vi "Get All PDP Data.vi"(0 "Power Distribution Panel (0)":u8, 11 "error in":errorcluster) -> (6 "PDP Data":T1, 15 "error out":errorcluster)   [LabVIEW 2014]
doc: "Returns the currents of the Power Distribution Panel (PDP) channels."
uses:
  PDP Data.ctl
  <vilib>/Rock Robotics/WPI/CAN/PDP/WPI_CAN_PDPGlobalOps.ctl
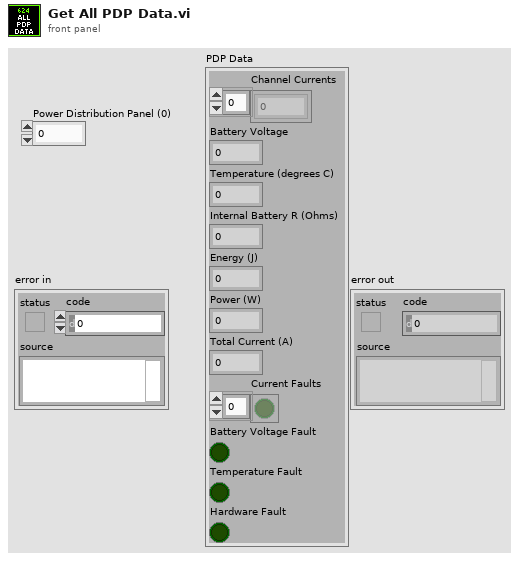
[diagram p1: front panel]
types:
  T1 = typedef "PDP Data.ctl" = cluster{"Channel Currents":dbl[], "Battery Voltage":dbl, "Temperature (degrees C)":dbl, "Internal Battery R (Ohms)":dbl, "Energy (J)":dbl, "Power (W)":dbl, "Total Current (A)":dbl, "Current Faults":bool[], "Battery Voltage Fault":bool, "Temperature Fault":bool, "Hardware Fault":bool}
  T2 = typedef "WPI_CAN_PDPGlobalOps.ctl" = enum16{"Write After Receive 0-5", "Write After Receive 6-11", "Write After Receive 12-15", "Write After Receive Energy", "Get All", "Get Commands", "Write Clear Sticky Faults Command", "Write Reset Energy Command", "Write Tare Currents Command", "Write Error", "Write After Receive Faults"}
  T3 = typedef "WPI_CAN_PDPGetAll.ctl" = cluster{"Channel Currents":dbl[], "Battery Voltage":dbl, "Temperature (degrees C)":dbl, "Internal Battery R (Ohms)":dbl, "Energy (J)":dbl, "Power (W)":dbl, "Total Current (A)":dbl, "CAN Error":errorcluster, "Current Faults":bool[], "Battery Voltage Fault":bool, "Temperature Fault":bool, "Hardware Fault":bool}
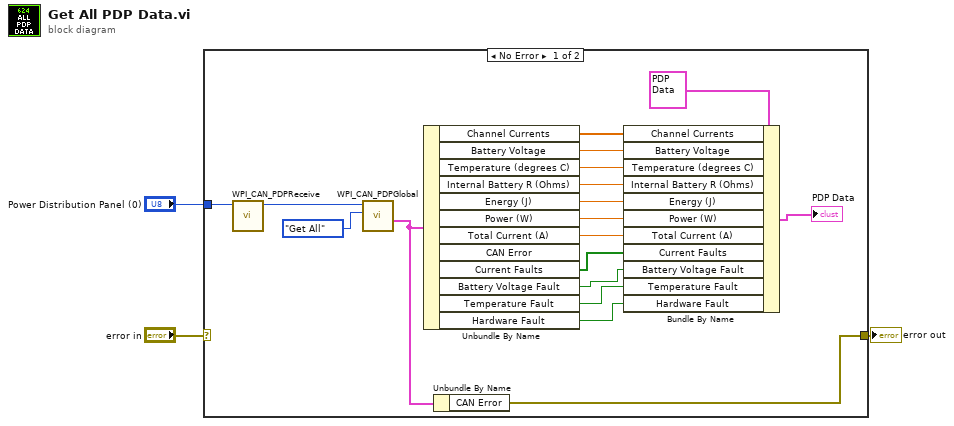
[diagram p0: block diagram]
diagram:
  n1 = case shown="No Error" "error in" {
    selector: "error in" -> [_ w22]
    tunnel: [w18 w22] -> w2
    tunnel: "Power Distribution Panel (0)" -> [w20 _]
    frame No Error {
      n2 = call <vilib>:"WPI_CAN_PDPReceive.vi"("Power Distribution Panel (0)"=w20) -> ("Power Distribution Panel Out"=w21:u8)  [unwired: 10 in]
      n3 = call <vilib>:"WPI_CAN_PDPGlobal.vi"("Operation"=WPI_CAN_PDPGlobalOps."Get All", "Power Distribution Panel (0)"=w21) -> ("Get All"=w17:T3)  [unwired: 7 in, 2 out]
      n4 = Unbundle By Name(w17) -> ("Channel Currents"=w14:dbl[], "Battery Voltage"=w13:dbl, "Temperature (degrees C)"=w12:dbl, "Internal Battery R (Ohms)"=w11:dbl, "Energy (J)"=w10:dbl, "Power (W)"=w9:dbl, "Total Current (A)"=w8:dbl, "Current Faults"=w7:bool[], "Battery Voltage Fault"=w6:bool, "Temperature Fault"=w5:bool, "Hardware Fault"=w4:bool)  [unwired: 1 out]
      n5 = Unbundle By Name(w17) -> ("CAN Error"=w18:errorcluster)
      n6 = Bundle By Name(cluster=T1 {"Channel Currents"=[], "Battery Voltage"=0.0, "Temperature (degrees C)"=0.0, "Internal Battery R (Ohms)"=0.0, "Energy (J)"=0.0, "Power (W)"=0.0, "Total Current (A)"=0.0, "Current Faults"=[], "Battery Voltage Fault"=FALSE, "Temperature Fault"=FALSE, "Hardware Fault"=FALSE} ("PDP Data"), "Channel Currents"=w14, "Battery Voltage"=w13, "Temperature (degrees C)"=w12, "Internal Battery R (Ohms)"=w11, "Energy (J)"=w10, "Power (W)"=w9, "Total Current (A)"=w8, "Current Faults"=w7, "Battery Voltage Fault"=w6, "Temperature Fault"=w5, "Hardware Fault"=w4) -> (→"PDP Data":T1)
    }
    frame Error {
    }
  }
  "error out" <- w2
